vi "DSF.Engine.Transceiver Loader.Load Transceiver Classes.vi"(8 "error in (no error)":errorcluster, 11 "Transceiver Loader in":refnum<class "DSF.Engine.Transceiver Loader.lvclass">) -> (0 "error out":errorcluster, 2 "Transceivers":refnum<class "DSF.Engine.Transceiver.lvclass">[](array[class]), 3 "Transceiver Loader out":refnum<class "DSF.Engine.Transceiver Loader.lvclass">)   [LabVIEW 2017, in "Data Sharing Framework Engine.lvlib" / "DSF.Engine.Transceiver Loader.lvclass"]
uses:
  DSF.Engine.Transceiver Loader.lvclass
  DSF.Engine.Transceiver.lvclass
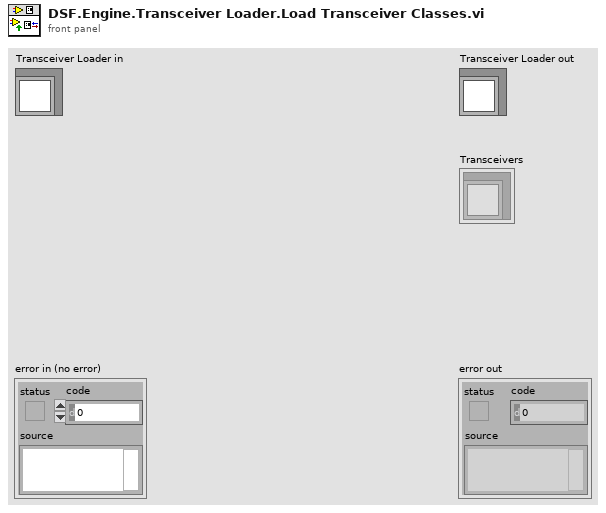
[diagram p1: front panel]
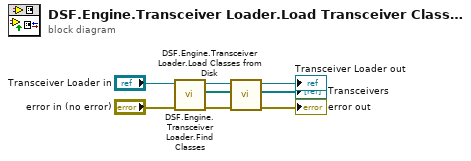
[diagram p0: block diagram]
diagram:
  n1 = call "DSF.Engine.Transceiver Loader.Find Classes.vi"("error in (no error)"="error in (no error)", "Transceiver Loader in"="Transceiver Loader in") -> ("error out"=w6:errorcluster, "class paths"=w1:path[], "Transceiver Loader out"=w5:refnum<class "DSF.Engine.Transceiver Loader.lvclass">)  [unwired: 7 in]
  n2 = call "DSF.Engine.Transceiver Loader.Load Classes from Disk.vi"("error in (no error)"=w6, "class paths"=w1, "Transceiver Loader in"=w5) -> ("error out"=→"error out":errorcluster, "Transceivers"=→"Transceivers":refnum<class "DSF.Engine.Transceiver.lvclass">[], "Transceiver Loader out"=→"Transceiver Loader out":refnum<class "DSF.Engine.Transceiver Loader.lvclass">)  [unwired: 6 in]
